vi "NMRFMTCP2.vi"() -> ()   [LabVIEW 2013]
uses:
  <vilib>/Analysis/2dsp.llb/Power Spectrum (DBL).vi
  <vilib>/Analysis/NI_AALBase.lvlib
  <vilib>/Analysis/NI_AALPro.lvlib
panel:
  in  "IP Address":string="192.168.1.162"
  out "FFT Vrms":dbl[](graph)=[0.00491288724422558, 0.004766817799000612, 0.0028347968420014504, 0.00032948259885015016, 0.0007684180461732006, 0.00013461327874688263, 0.0007676915015052642, 0.0003124754799638557, 0.0005542319259414395, 0.0001528235231485258, 0.00012209918011686725, 0.00029999774448873486, 0.00035510982656143626, 0.00012034427911409962, 0.0002622313132652784, 0.00023394631136381392, 0.0004552768836821714, 0.00022947008023570077, 0.00016515382589768265, 0.000533723018673728, 0.00010203360529099216, 0.0001782801878483863, 0.0002684368673757001, 0.0002911776068689857, 2.97512444146063e-05, 0.00025573572949118105, 0.000173696754425059, 0.00021335007604465696, 0.00017095685621183472, 0.0002577887953281745, 7.818504622882473e-05, 0.00023607164482181798, 5.356981939781055e-05, 5.6629280526844514e-05, 8.16922787821161e-05, 0.00013697739713077928, 8.53294702102032e-05, 0.00013239362335425582, 0.00024243690700732426, 0.00033894985716797956, 0.0002711681574789461, 0.0002004623280762697, 0.00018846229233582265, 0.00019547824500197274, 0.0002613330782674258, 0.00017358867498694735, 0.0002622611618019136, 0.00015461352411319805, 2.3075049750455087e-05, 0.00015362372956081617, 0.00018087844752279824, 0.00018087844752279824, 0.00015362372956081617, 2.3075049750455087e-05, 0.00015461352411319805, 0.0002622611618019136, 0.00017358867498694735, 0.0002613330782674258, 0.00019547824500197274, 0.00018846229233582265, 0.0002004623280762697, 0.0002711681574789461, 0.00033894985716797956, 0.00024243690700732426, 0.00013239362335425582, 8.53294702102032e-05, 0.00013697739713077928, 8.16922787821161e-05, 5.6629280526844514e-05, 5.356981939781055e-05, 0.00023607164482181798, 7.818504622882473e-05, 0.0002577887953281745, 0.00017095685621183472, 0.00021335007604465696, 0.000173696754425059, 0.00025573572949118105, 2.97512444146063e-05, 0.0002911776068689857, 0.0002684368673757001, 0.0001782801878483863, 0.00010203360529099216, 0.000533723018673728, 0.00016515382589768265, 0.00022947008023570077, 0.0004552768836821714, 0.00023394631136381392, 0.0002622313132652784, 0.00012034427911409962, 0.00035510982656143626, 0.00029999774448873486, 0.00012209918011686725, 0.0001528235231485258, 0.0005542319259414395, 0.0003124754799638557, 0.0007676915015052642, 0.00013461327874688263, 0.0007684180461732006, 0.00032948259885015016, 0.0028347968420014504, 0.004766817799000612]
  out "NMR Ave Graph":cluster{dbl, "Step Width (MHz)":dbl, dbl[][]}(graph)
  in  "GPIB Addr (28)":refnum<visa-resource-name>="GPIB0::28::INSTR"
  out "Pedestal (V)":dbl=2.049694229166664 format="%_2g"
  in  "Open Global Panel":bool=TRUE
  out "Peak center (MHz)":sgl=213.36436 format="%.3f"
  out "Telnet error out":errorcluster
  out "+3.3V supply":dbl=3.294 format="%_4g"
  out "Temp (C)":dbl=28.25 format="%_4g"
  out "RF OK":bool=TRUE
  out "Peak area (V-MHz)":sgl=0.00055034726 format="%.5f"
  out "NMR Graph + Fit":cluster{cluster{dbl, "Numeric":dbl}[]}[](graph)=[{[{213.31, "Numeric"=0.001874778333337268}, {213.311, "Numeric"=0.0018717783333515037}, {213.312, "Numeric"=0.0008088383333650917}, {213.313, "Numeric"=0.006685958333297215}, {213.314, "Numeric"=0.003503138333311284}, {213.315, "Numeric"=0.0002603783333250398}, {213.316, "Numeric"=-0.0030423216666624064}, {213.317, "Numeric"=0.0015950383333502849}, {213.318, "Numeric"=-0.0028275416666381226}, {213.319, "Numeric"=-0.0003100616666973366}, {213.32, "Numeric"=-0.0008525216666850355}, {213.321, "Numeric"=-0.003454921666673272}, {213.322, "Numeric"=-0.004117261666662042}, {213.323, "Numeric"=-0.003839541666651236}, {213.324, "Numeric"=-0.002621761666640854}, {213.325, "Numeric"=-0.004463921666691739}, {213.326, "Numeric"=-0.007366021666681544}, {213.327, "Numeric"=-0.008328061666670994}, {213.328, "Numeric"=-0.007350041666661866}, {213.329, "Numeric"=-0.008431961666652832}, {213.33, "Numeric"=-0.004573821666644662}, {213.331, "Numeric"=-0.004775621666686547}, {213.332, "Numeric"=-0.002037361666678006}, {213.333, "Numeric"=-0.0013590416666695582}, {213.334, "Numeric"=0.0002593383333384658}, {213.335, "Numeric"=0.0008177783333453981}, {213.336, "Numeric"=-0.002683721666647987}, {213.337, "Numeric"=-0.0002451616666823142}, {213.338, "Numeric"=-0.0028665416666751042}, {213.339, "Numeric"=0.003452138333332133}, {213.34, "Numeric"=0.0027108783333380515}, {213.341, "Numeric"=-0.0020903216666563473}, {213.342, "Numeric"=4.853833334861335e-05}, {213.343, "Numeric"=0.0001274583333228385}, {213.344, "Numeric"=0.00014643833332828038}, {213.345, "Numeric"=-0.0008945216666664813}, {213.346, "Numeric"=0.001004578333337669}, {213.347, "Numeric"=0.007843738333341399}, {213.348, "Numeric"=0.0046229583333445845}, {213.349, "Numeric"=0.00834223833332759}, {213.35, "Numeric"=0.011001578333331263}, {213.351, "Numeric"=0.01360097833333418}, {213.352, "Numeric"=0.015140438333337336}, {213.353, "Numeric"=0.009619958333339174}, {213.354, "Numeric"=0.008039538333340701}, {213.355, "Numeric"=0.014399178333332152}, {213.356, "Numeric"=0.018698878333334168}, {213.357, "Numeric"=0.017938638333335533}, {213.358, "Numeric"=0.020118458333336253}, {213.359, "Numeric"=0.015238338333336543}, {213.36, "Numeric"=0.018298278333336526}, {213.361, "Numeric"=0.02129827833333664}, {213.362, "Numeric"=0.020238338333336436}, {213.363, "Numeric"=0.024118458333336257}, {213.364, "Numeric"=0.014938638333335419}, {213.365, "Numeric"=0.02169887833333428}, {213.36599999999999, "Numeric"=0.02039917833333238}, {213.367, "Numeric"=0.020039538333340712}, {213.368, "Numeric"=0.021619958333339184}, {213.369, "Numeric"=0.023140438333337343}, {213.37, "Numeric"=0.019600978333334407}, {213.371, "Numeric"=0.02000157833333116}, {213.37199999999999, "Numeric"=0.015342238333327707}, {213.373, "Numeric"=0.013622958333344481}, {213.374, "Numeric"=0.012843738333341292}, {213.375, "Numeric"=0.01200457833333779}, {213.376, "Numeric"=0.014105478333333643}, {213.377, "Numeric"=0.005146438333328618}, {213.378, "Numeric"=0.004127458333322842}, {213.379, "Numeric"=0.005048538333348507}, {213.38, "Numeric"=0.002909678333343546}, {213.381, "Numeric"=0.006710878333338055}, {213.382, "Numeric"=0.006452138333331803}, {213.383, "Numeric"=0.01313345833332491}, {213.384, "Numeric"=0.007754838333317693}, {213.385, "Numeric"=0.0033162783333522405}, {213.386, "Numeric"=0.004817778333345402}, {213.387, "Numeric"=0.004259338333338469}, {213.388, "Numeric"=0.005640958333330115}, {213.389, "Numeric"=0.0019626383333219977}, {213.39, "Numeric"=-0.0007756216666865434}, {213.391, "Numeric"=-0.0015738216666445481}, {213.392, "Numeric"=-0.0024319616666530486}, {213.393, "Numeric"=-0.0023500416666615287}, {213.394, "Numeric"=-0.0023280616666712106}, {213.395, "Numeric"=-0.002366021666681206}, {213.396, "Numeric"=-0.0014639216666920696}, {213.397, "Numeric"=-0.0006217616666410741}, {213.398, "Numeric"=0.002160458333348547}, {213.399, "Numeric"=-0.00011726166666203852}, {213.4, "Numeric"=0.0015450783333266216}, {213.401, "Numeric"=-0.0018525216666849253}, {213.402, "Numeric"=-0.0013100616666972265}, {213.403, "Numeric"=0.001172458333361881}, {213.404, "Numeric"=0.0015950383333502849}, {213.405, "Numeric"=0.0009576783333375971}, {213.406, "Numeric"=-0.0007396216666748501}, {213.407, "Numeric"=0.0015031383333115045}, {213.408, "Numeric"=0.0036859583332971013}, {213.409, "Numeric"=0.0028088383333653155}, {213.41, "Numeric"=0.0028717783333513935}]}]
  out "# Good Spectra":i32=100
  out "Pedestal OK":bool=TRUE
  out "Sweep #":i32=18
  out "1st Sweep":bool
  out "ADC volts OK":bool=TRUE
  out "Peak Height Distribution":cluster{"Y":dbl[], "Y":dbl[]}[](graph)=[{"Y"=[0.020157212566669552, 0.020308414366669556, 0.02045961616666956, 0.02061081796666956, 0.020762019766669564, 0.020913221566669568, 0.02106442336666957, 0.021215625166669572, 0.021366826966669573, 0.021518028766669577, 0.02166923056666958, 0.02182043236666958, 0.021971634166669585, 0.02212283596666959, 0.02227403776666959, 0.022425239566669593, 0.022576441366669597, 0.022727643166669597, 0.0228788449666696, 0.0230300467666696, 0.023181248566669605, 0.02333245036666961, 0.02348365216666961, 0.023634853966669613, 0.023786055766669617, 0.023937257566669617, 0.02408845936666962, 0.024239661166669625, 0.024390862966669626, 0.02454206476666963, 0.024693266566669633, 0.024844468366669634, 0.024995670166669638, 0.025146871966669638, 0.025298073766669642, 0.025449275566669646, 0.025600477366669646, 0.02575167916666965, 0.025902880966669654, 0.026054082766669654, 0.026205284566669658, 0.026356486366669662, 0.026507688166669662, 0.026658889966669666, 0.026810091766669666, 0.02696129356666967, 0.027112495366669674, 0.027263697166669675, 0.02741489896666968, 0.027566100766669682, 0.027717302566669683, 0.027868504366669686, 0.02801970616666969, 0.02817090796666969, 0.028322109766669695, 0.0284733115666697, 0.0286245133666697, 0.028775715166669703, 0.028926916966669703, 0.029078118766669707, 0.02922932056666971, 0.02938052236666971, 0.029531724166669715, 0.02968292596666972, 0.02983412776666972, 0.029985329566669723, 0.030136531366669727, 0.030287733166669727, 0.03043893496666973, 0.03059013676666973, 0.030741338566669735, 0.03089254036666974, 0.03104374216666974, 0.031194943966669744, 0.03134614576666975, 0.03149734756666975, 0.03164854936666975, 0.031799751166669755, 0.031950952966669756, 0.032102154766669756, 0.032253356566669764, 0.032404558366669764, 0.032555760166669764, 0.03270696196666977, 0.03285816376666977, 0.03300936556666977, 0.03316056736666978, 0.03331176916666978, 0.03346297096666978, 0.03361417276666979, 0.03376537456666979, 0.03391657636666979, 0.034067778166669796, 0.034218979966669796, 0.0343701817666698, 0.034521383566669804, 0.034672585366669804, 0.034823787166669805, 0.03497498896666981, 0.03512619076666981], "Y"=[1.0, 0.0, 0.0, 1.0, 0.0, 0.0, 1.0, 0.0, 0.0, 1.0, 0.0, 0.0, 2.0, 0.0, 2.0, 0.0, 0.0, 0.0, 0.0, 0.0, 1.0, 2.0, 2.0, 1.0, 3.0, 1.0, 1.0, 1.0, 2.0, 0.0, 0.0, 0.0, 0.0, 0.0, 3.0, 1.0, 2.0, 3.0, 2.0, 1.0, 4.0, 1.0, 2.0, 2.0, 0.0, 1.0, 3.0, 0.0, 4.0, 2.0, 2.0, 0.0, 1.0, 7.0, 5.0, 2.0, 1.0, 0.0, 2.0, 3.0, 1.0, 1.0, 3.0, 1.0, 2.0, 0.0, 2.0, 2.0, 1.0, 0.0, 1.0, 0.0, 2.0, 0.0, 1.0, 0.0, 1.0, 0.0, 1.0, 0.0, 0.0, 0.0, 0.0, 0.0, 0.0, 0.0, 1.0, 0.0, 0.0, 2.0, 0.0, 0.0, 1.0, 0.0, 0.0, 0.0, 0.0, 0.0, 0.0, 1.0]}]
  out "S/N":dbl=8.889914894885075 format="%_3g"
  out "Peak mean (V)":dbl=0.027208529933335814 format="%_4g"
  out "Pedestal Diff (V)":sgl=0.00362787 format="%.3f"
  out "Peak amp (V)":sgl=0.024118459 format="%.3f"
  out "SMT error out":errorcluster
  out "Peak RMS (mV)":dbl format="%.3f"
  # "E1039 NMR Panel"
  # "Results"
  # "A\nv\ne\nr\na\ng\ne\ns"
  # "S\nw\ne\ne\np"
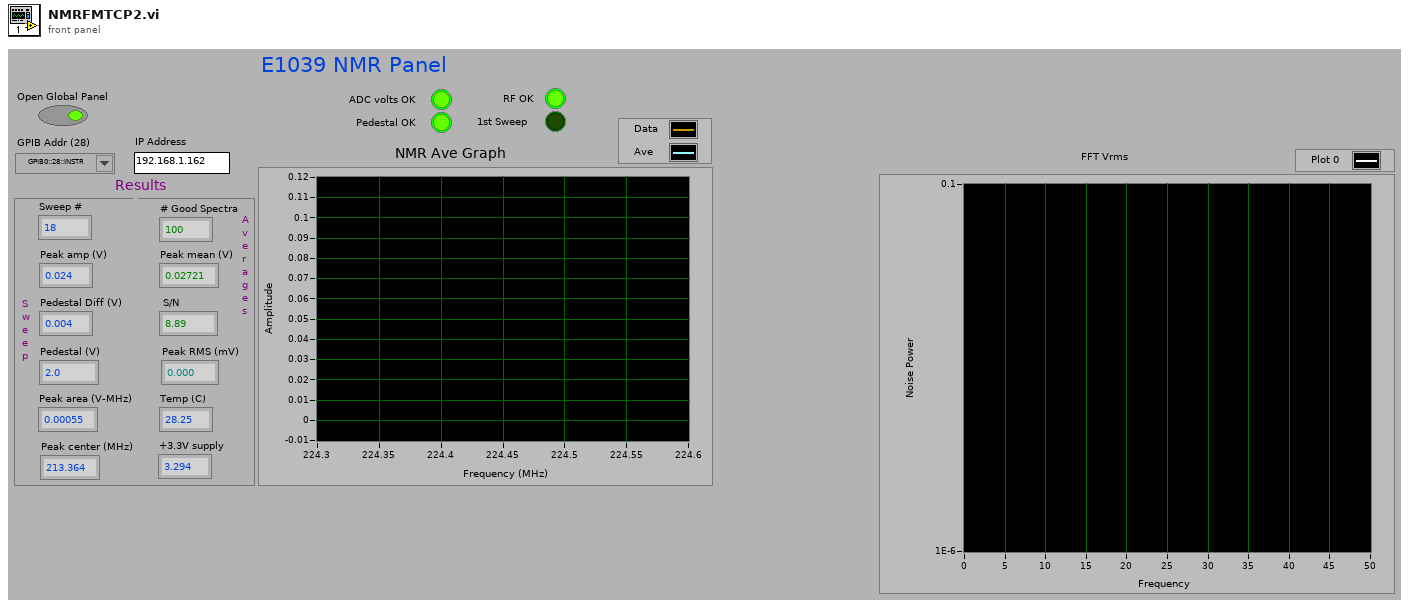
[diagram p1: front panel]
types:
  T1 = enum32{"Invalid", "Standard", "Closed", "Hidden", "Minimized", "Maximized"}
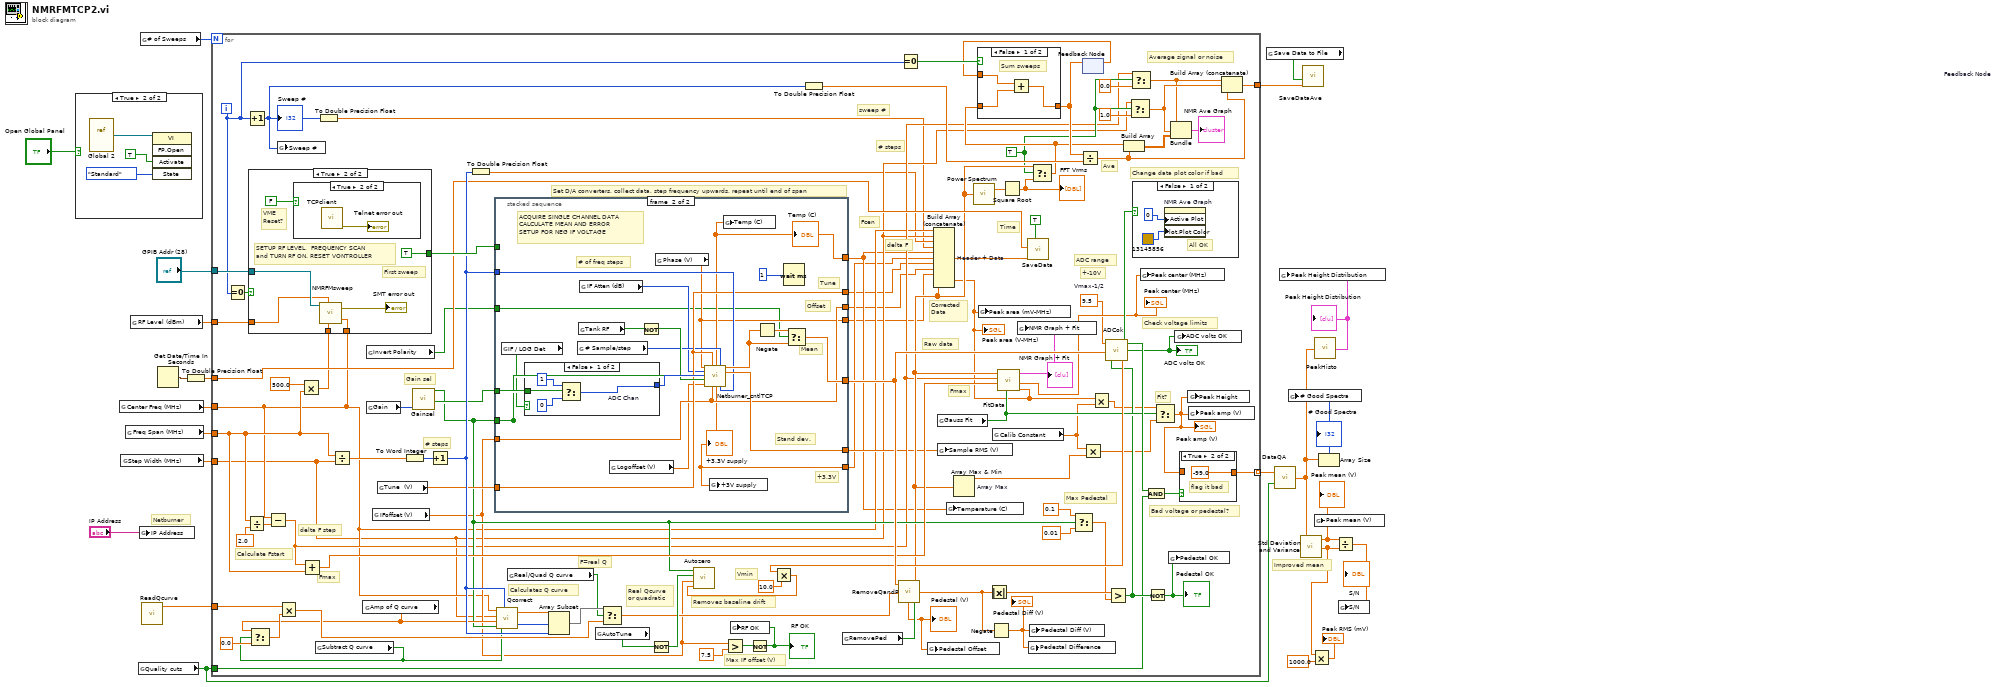
[diagram p0: block diagram]
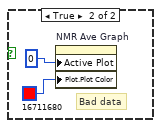
[diagram p4: hidden frame]
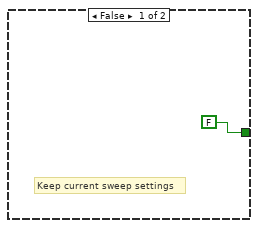
[diagram p6: hidden frame]
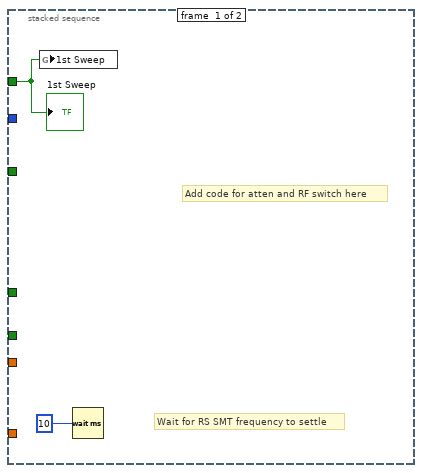
[diagram p8: hidden frame]
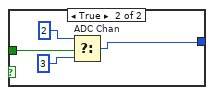
[diagram p9: hidden frame]
diagram:
  # "Netburner"
  # "Improved mean"
  n1 = case shown="True" "Open Global Panel" {
    frame False {
    }
    frame True {
      n2 = vi-ref "Global 2.vi"() -> (w26:refnum<vi>)
      n3 = invoke class="VI" method="FP.Open"(reference=w26, "Activate"=TRUE, "State"=T1."Standard") -> ()  [unwired: 2 in, 5 out]
    }
  }
  n4 = global read "Global 2.vi" "Center Freq (MHz)"() -> (w18:dbl)
  n5 = global read "Global 2.vi" "Step Width (MHz)"() -> (w16:dbl)
  n6 = global read "Global 2.vi" "Freq Span (MHz)"() -> (w17:dbl)
  n7 = global read "Global 2.vi" "RF Level (dBm)"() -> (w19:dbl)
  n8 = global read "Global 2.vi" "Quality cuts"() -> (w15:bool)
  n9 = global write "Global 2.vi" "IP Address"("IP Address") -> ()
  n10 = global read "Global 2.vi" "# of Sweeps"() -> (w20:i32)
  n11 = call "ReadQcurve.vi"() -> ("Array"=w5:dbl[])  [unwired: 2 in]
  n12 = Get Date/Time In Seconds() -> (seconds since 1Jan1904=w21:timestamp)
  n13 = To Double Precision Float(number=w21) -> (double precision float=w6:dbl)
  n14 = for {
    N: w20 -> [_]
    tunnel: [w115] -> w23 mode=indexing
    tunnel: w15 -> [w74]
    tunnel: w18 -> [w41]
    tunnel: w17 -> [w54]
    tunnel: w16 -> [w40]
    tunnel: "GPIB Addr (28)" -> [w110]
    tunnel: w19 -> [w109]
    tunnel: w6 -> [w107]
    tunnel: w5 -> [w99]
    tunnel: [w60] -> w8
    i -> [w56]
    w46 = TRUE
    w68 = 9.5  # Vmax-1/2
    # "Average signal or noise"
    # "Check voltage limits"
    # "Ave"
    # "Max Pedestal"
    # "Gain sel"
    # "F=real Q"
    # "Real Qcurve\nor quadratic"
    # "+-10V"
    # "Change data plot color if bad"
    # "Max IF offset (V)"
    # "Fmax"
    # "Fit?"
    # "Fmax"
    # "Time"
    # "Vmin"
    # "Raw data"
    # "Corrected\nData"
    # "Fcen"
    # "delta F"
    # "# steps"
    # "ADC range"
    # "sweep #"
    # "Set D/A converters, collect data, step frequency upwards, repeat until end of span"
    # "Calculates Q curve"
    # "Removes baseline drift"
    # "Bad voltage or pedestal?"
    # "# steps"
    # "Calculate Fstart"
    # "delta F step"
    n15 = Equal To 0?(x=w56) -> (x = 0?=w117:bool)
    n16 = Divide(x=w54, y=sgl 2.0) -> (x/y=w121:dbl)
    n17 = Increment(x=w56) -> (x+1=w72:i32)
    "Sweep #" <- w72
    n18 = Subtract(x=w41, y=w121) -> (x-y=w44:dbl)
    n19 = global write "Global 2.vi" "Sweep #"(w72) -> ()
    n20 = Multiply(x=500.0, y=w54) -> (x*y=w53:dbl)
    n21 = case shown="True" w117 {
      tunnel: w41 -> [_ w140]
      tunnel: w53 -> [_ w141]
      tunnel: [FALSE TRUE] -> w116
      tunnel: w110 -> [_ w137]
      tunnel: w109 -> [_ w136]
      frame False {
        # "Keep current sweep settings"
      }
      frame True {
        # "VME\nReset?"
        # "First sweep"
        # "SETUP RF LEVEL,  FREQUENCY SCAN\nand TURN RF ON. RESET VONTROLLER"
        n22 = case shown="True" FALSE {
          frame False {
          }
          frame True {
            n23 = call "TCPclient.vi"() -> ("Telnet error"=→"Telnet error out":errorcluster)  [unwired: 4 in, 3 out]
          }
        }
        n24 = call "NMRFMsweep.vi"("Center Freq (MHz)"=w140, "Freq Span (kHz)"=w141, "RF Level (dBm)"=w136, "GPIB Addr (28)"=w137) -> ("error out"=→"SMT error out":errorcluster)  [unwired: 3 in]
      }
    }
    n25 = Add(x=w44, y=w54) -> (x+y=w104:dbl)
    n26 = global read "Global 2.vi" "Subtract Q curve"() -> (w90:bool)
    n27 = To Double Precision Float(number=w72) -> (double precision float=w38:dbl)
    n28 = Divide(x=w54, y=w40) -> (x/y=w123:dbl)
    n29 = global read "Global 2.vi" "Amp of Q curve"() -> (w91:dbl)
    n30 = Select(t=w91, s=w90, f=0.0) -> (s? t:f=w96:dbl)
    n31 = Multiply(x=w99, y=w96) -> (x*y=w98:dbl[])
    n32 = global read "Global 2.vi" "Invert Polarity"() -> (w32:bool)
    n33 = global read "Global 2.vi" "Gain"() -> (w63:enum16{"LOW", "HI", "MAX"})
    n34 = global read "Global 2.vi" "IFoffset (V)"() -> (w59:dbl)
    n35 = global read "Global 2.vi" "Tune  (V)"() -> (w92:dbl)
    n36 = To Word Integer(number=w123) -> (16bit integer=w120:i16)
    n37 = call "Gainsel.vi"("Gain"=w63) -> ("LO"=w64:bool, "MAX"=w62:bool)  [unwired: 1 out]
    n38 = Increment(x=w120) -> (x+1=w111:i16)
    n39 = To Double Precision Float(number=w111) -> (double precision float=w39:dbl)
    n40 = stacked-sequence {
      tunnel: [_ w160] -> w42
      tunnel: [_ w164] -> w108
      tunnel: w111 -> [_ w158]
      tunnel: w59 -> [_ w155]
      tunnel: w64 -> [_ w162]
      tunnel: w116 -> [w143 _]
      tunnel: w92 -> [_ w156]
      tunnel: [_ w148] -> w37
      tunnel: [_ w147] -> w36
      tunnel: [_ w156] -> w35
      tunnel: [_ w155] -> w34
      tunnel: [_ w154] -> _
      tunnel: w62 -> [_ w154]
      tunnel: [_ w146] -> w33
      tunnel: w32 -> [_ w145]
      frame #0 {
        # "Add code for atten and RF switch here"
        # "Wait for RS SMT frequency to settle"
        n41 = global write "Global 2.vi" "1st Sweep"(w143) -> ()
        n42 = Wait (ms)(milliseconds to wait=10) -> ()  [unwired: 1 out]
        "1st Sweep" <- w143
      }
      frame #1 {
        # "+3.3V"
        # "Offset"
        # "Tune"
        # "Stand dev."
        # "Mean"
        # "ACQUIRE SINGLE CHANNEL DATA\nCALCULATE MEAN AND ERROR\nSETUP FOR NEG IF VOLTAGE"
        # "# of freq steps"
        n43 = global read "Global 2.vi" "IF / LOG Det"() -> (w152:bool)
        n44 = case shown="False" w152 {
          tunnel: w162 -> [w169 w170]
          tunnel: [w166 w171] -> w159
          frame False {
            n45 = Select "ADC Chan"(t=1, s=w169, f=0) -> (s? t:f=w166:i32)
          }
          frame True {
            n46 = Select "ADC Chan"(t=2, s=w170, f=3) -> (s? t:f=w171:i32)
          }
        }
        n47 = global read "Global 2.vi" "# Sample/step"() -> (w150:i32)
        n48 = global read "Global 2.vi" "Tank RF"() -> (w151:bool)
        n49 = global read "Global 2.vi" "IF Atten (dB)"() -> (w149:i8)
        n50 = global read "Global 2.vi" "Logoffset (V)"() -> (w153:dbl)
        n51 = Not(x=w151) -> (.not. x?=w157:bool)
        n52 = global read "Global 2.vi" "Phase (V)"() -> (w146:dbl)
        n53 = call "Netburner_cntlTCP.vi"("Phase Volt"=w146, "Tune Volt"=w156, "# Data"=w150, "IF Atten (dB)"=w149, "NMR ADC"=w159, "Hi Gain"=w154, "Tank RF"=w157, "LogOff Volt"=w153, "IFOff Volt"=w155, "# f steps"=w158) -> ("Temp (C)"=w148:dbl, "ADC value"=w161:dbl[], "ADC Std Dev"=w160:dbl, "Volts"=w147:dbl)  [unwired: 2 out]
        "Temp (C)" <- w148
        "+3.3V supply" <- w147
        n54 = global write "Global 2.vi" "+3V supply"(w147) -> ()
        n55 = global write "Global 2.vi" "Temp (C)"(w148) -> ()
        n56 = Negate(x=w161) -> (-x=w163:dbl[])
        n57 = Wait (ms)(milliseconds to wait=1) -> ()  [unwired: 1 out]
        n58 = Select(t=w163, s=w145, f=w161) -> (s? t:f=w164:dbl[])
      }
    }
    n59 = call "Qcorrect.vi"("Subtract Q curve"=w90, "Nstep"=w111, "Max Gain"=w62, "Amp of Q curve"=w91, "Step Width (MHz)"=w40, "Center Freq (MHz)"=w41) -> ("Start"=w118:i32, "Array"=w119:dbl[])
    n60 = global read "Global 2.vi" "Real/Quad Q curve"() -> (w89:bool)
    n61 = Array Subset "Array Subset"(array=w119, index=w118, length=w111) -> (w101:dbl[])
    n62 = global read "Global 2.vi" "AutoTune"() -> (w87:bool)
    n63 = Select(t=w101, s=w89, f=w98) -> (s? t:f=w100:dbl[])
    n64 = Not(x=w87) -> (.not. x?=w102:bool)
    n65 = Greater?(x=w59, y=7.5) -> (0:w105:bool)
    n66 = Not(x=w105) -> (.not. x?=w83:bool)
    "RF OK" <- w83
    n67 = global write "Global 2.vi" "RF OK"(w83) -> ()
    n68 = To Double Precision Float(number=w72) -> (double precision float=w66:dbl)
    n69 = global read "Global 2.vi" "RemovePed"() -> (w88:bool)
    n70 = call "RemoveQandP.vi"("Subtract Ped?"=w88, "Qcurve"=w100, "Raw data"=w108) -> ("Ped L-R"=w112:dbl, "Corrected data"=w50:dbl[], "Ped Offfset"=w78:dbl)
    "Pedestal (V)" <- w78
    n71 = Equal To 0?(x=w56) -> (x = 0?=w71:bool)
    n72 = global write "Global 2.vi" "Pedestal Offset"(w78) -> ()
    n73 = global read "Global 2.vi" "Gauss Fit"() -> (w86:bool)
    n74 = global write "Global 2.vi" "Sample RMS (V)"(w42) -> ()
    n75 = global write "Global 2.vi" "Temperature (C)"(w37) -> ()
    n76 = Array Max & Min "Array Max"(array=w50) -> (max value=w31:dbl)  [unwired: 3 out]
    n77 = call-poly <vilib>:"Power Spectrum.vi"("X"=w50) -> ("Power Spectrum"=w55:dbl[])  [unwired: 1 out]
    n78 = Absolute Value ("Abs Value")(x=w112) -> (abs(x)=w113:dbl)
    n79 = Negate(x=w112) -> (-x=w79:dbl)
    "Pedestal Diff (V)" <- w79
    n80 = global read "Global 2.vi" "Calib Constant"() -> (w28:dbl)
    n81 = call "FitData.vi"("Fit?"=w86, "Fmax"=w104, "Fmin"=w44, "Yarray"=w50) -> ("Peak Area (mV-MHz)"=w29:dbl, "Center Freq (MHz)"=w82:dbl, "NMR Graph + Fit"=w80:cluster{cluster{dbl, "Numeric":dbl}[]}[])  [unwired: 2 out]
    "NMR Graph + Fit" <- w80
    "Peak area (V-MHz)" <- w29
    "Peak center (MHz)" <- w82
    n82 = Build Array (concatenate) "Header + Data"(w41, w40, w39, w38, w37, w36, w35, w34, w33, w29, w50) -> (w57:dbl[])
    n83 = global write "Global 2.vi" "Peak area (mV-MHz)"(w29) -> ()
    n84 = Square Root(x=w55) -> (sqrt(x)=w51:dbl[])
    "FFT Vrms" <- w51
    n85 = global write "Global 2.vi" "NMR Graph + Fit"(w80) -> ()
    n86 = call "SaveData.vi"("Array"=w57, "Save Data to File"=TRUE, "Ext time (sec)"=w107) -> ()  [unwired: 1 out]
    n87 = global write "Global 2.vi" "Pedestal Difference"(w79) -> ()
    n88 = global write "Global 2.vi" "Pedestal Diff (V)"(w79) -> ()
    n89 = Select(t=w50, s=w46, f=w51) -> (s? t:f=w49:dbl[])
    n90 = Select(t=0.1, s=w62, f=0.01) -> (s? t:f=w73:dbl)
    n91 = feedback #1 "Feedback Node"() -> (w70:dbl[])  [unwired: 1 in]
    n92 = case shown="False" w71 {
      tunnel: w49 -> [w125 w127]
      tunnel: [w124 w127] -> w67
      tunnel: w70 -> [w126 _]
      frame False {
        # "Sum sweeps"
        n93 = Add(x=w126, y=w125) -> (x+y=w124:dbl[])
      }
      frame True {
        # "Initialize"
      }
    }
    n94 = Divide(x=w67, y=w66) -> (x/y=w61:dbl[])
    n95 = feedback-in #1(w67) -> ()
    n96 = Multiply(x=w28, y=w31) -> (x*y=w30:dbl)
    n97 = Multiply(x=w29, y=w28) -> (x*y=w27:dbl)
    n98 = Greater?(x=w113, y=w73) -> (0:w75:bool)
    n99 = call "ADCok.vi"("PedOK"=w75, "Array"=w108, "Vmax-1/2"=w68) -> ("Vmin"=w95:dbl, "ADC voltages OK"=w85:bool, "Allok"=w103:bool)
    "ADC volts OK" <- w85
    n100 = Multiply(x=w95, y=10.0) -> (x*y=w93:dbl)
    n101 = call "Autozero.vi"("Vmin (V)"=w93, "IFoffset (V)"=w59, "Enable"=w102, "Max Gain"=w62) -> ()
    n102 = Build Array "Build Array"(w49, w61) -> (w65:dbl[][])
    n103 = Select(t=w40, s=w46, f=1.0) -> (s? t:f=w47:dbl)
    n104 = Select(t=w44, s=w46, f=0.0) -> (s? t:f=w43:dbl)
    n105 = case shown="False" w103 {
      frame False {
        # "All OK"
        n106 = property on="NMR Ave Graph" class="WFGraph (strict)"("Active Plot"=0, "Plot.Plot Color"=u32 13145856) -> ()  [unwired: 2 in, 2 out]
      }
      frame True {
        # "Bad data"
        n107 = property on="NMR Ave Graph" class="WFGraph (strict)"("Active Plot"=0, "Plot.Plot Color"=u32 16711680) -> ()  [unwired: 2 in, 2 out]
      }
    }
    n108 = global write "Global 2.vi" "Peak center (MHz)"(w82) -> ()
    n109 = And(x=w103, y=w74) -> (x .and. y?=w114:bool)
    n110 = Not(x=w75) -> (.not. x?=w84:bool)
    "Pedestal OK" <- w84
    n111 = Select(t=w27, s=w86, f=w30) -> (s? t:f=w81:dbl)
    "Peak amp (V)" <- w81
    n112 = global write "Global 2.vi" "Pedestal OK"(w84) -> ()
    n113 = Bundle(w43, "Step Width (MHz)"=w47, w65) -> (→"NMR Ave Graph":cluster{dbl, "Step Width (MHz)":dbl, dbl[][]})  [unwired: 1 in]
    n114 = global write "Global 2.vi" "ADC volts OK"(w85) -> ()
    n115 = case shown="True" w114 {
      tunnel: [w132 -99.0] -> w115
      tunnel: w81 -> [w132 _]
      frame False {
        # "Data OK"
      }
      frame True {
        # "flag it bad"
      }
    }
    n116 = global write "Global 2.vi" "Peak Height"(w81) -> ()
    n117 = global write "Global 2.vi" "Peak amp (V)"(w81) -> ()
    n118 = Build Array (concatenate) "Build Array"(w43, w47, w61) -> (w60:dbl[])
  }
  n119 = global read "Global 2.vi" "Save Data to File"() -> (w7:bool)
  n120 = call "DataQA.vi"("Quality cuts"=w15, "Data In"=w23) -> ("Data Out"=w22:dbl[])
  n121 = call <vilib>:"Std Deviation and Variance.vi"("X"=w22) -> ("mean"=w13:dbl, "standard deviation"=w2:dbl)  [unwired: 1 in, 1 out]
  "Peak mean (V)" <- w13
  n122 = call "SaveDataAve.vi"("Array"=w8, "Save Data to File"=w7) -> ()  [unwired: 1 in, 1 out]
  n123 = Multiply(x=w2, y=1000.0) -> (x*y=→"Peak RMS (mV)":dbl)
  n124 = call "PeakHisto.vi"("Data Out"=w22) -> ("XY Graph"=w11:cluster{"Y":dbl[], "Y":dbl[]}[])
  "Peak Height Distribution" <- w11
  n125 = global write "Global 2.vi" "Peak Height Distribution"(w11) -> ()
  n126 = global write "Global 2.vi" "Peak mean (V)"(w13) -> ()
  n127 = Array Size(array=w22) -> (size(s)=w12:i32)
  "# Good Spectra" <- w12
  n128 = global write "Global 2.vi" "# Good Spectra"(w12) -> ()
  n129 = Divide(x=w13, y=w2) -> (x/y=w14:dbl)
  "S/N" <- w14
  n130 = global write "Global 2.vi" "S/N"(w14) -> ()
